vi "Auto Filenames addon.vi"() -> (3 "SubOrdner":string)   [LabVIEW 2020, in "Linearisierung v2.lvlib" / "SpanEinstellungen.lvlib"]
uses:
  SpanEinstellungen.lvlib
  Aktion FGV Post Processing.ctl
  Allgemein/allgemeine Sub-VIs.lvlib
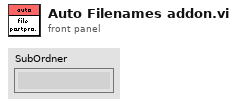
[diagram p1: front panel]
types:
  T1 = typedef "Linearisierung v2.lvlib/SpanEinstellungen.lvlib/Aktion FGV Post Processing.ctl" = enum16{"lesen", "set ref", "init", "reset", "enable", "disable", "filenames", "active", "comp", "filename index", "next", "first", "abort", "show"}
  T2 = typedef "Linearisierung v2.lvlib/SpanEinstellungen.lvlib/Postprocessing_Running_Indices.ctl" = cluster{"active postprocessing SPAN":i32, "active postprocessing SPAN Component":i32, "active postprocessing index":i32}
  T3 = cluster{"active Index Cluster out":T2, "last postprocessing SPAN ":bool}
  T4 = typedef "Pfad-Eingabefeld.ctl" = path
  T5 = cluster{"active SPAN Idx":i32, "Pfad .LIN Datei":T4}[]
  T6 = cluster{"active SPAN Idx":i32, "Pfad .LIN Datei":T4}
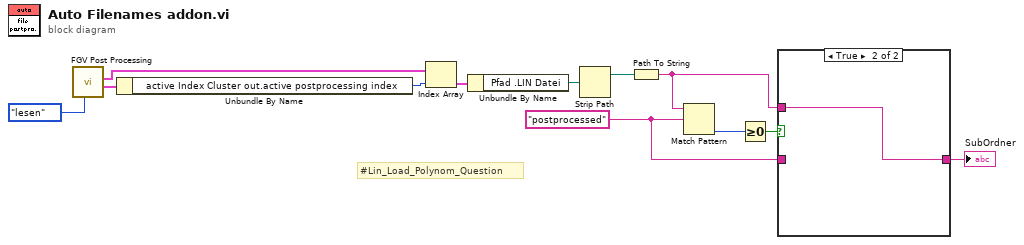
[diagram p0: block diagram]
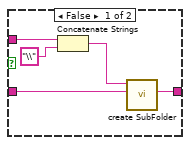
[diagram p2: hidden frame]
diagram:
  w2 = "postprocessed" ("String")
  # "#Lin_Load_Polynom_Question"
  n1 = call "FGV Post Processing.vi"("Aktion"=Aktion_FGV_Post_Processing."lesen") -> ("active Index Cluster out"=w6:T3, "filenemas Cluster Array"=w8:T5)  [unwired: 7 in, 2 out]
  n2 = Unbundle By Name(w6) -> ("active Index Cluster out.active postprocessing index"=w7:i32)
  n3 = Index Array(array=w8, index=w7) -> (element=w9:T6)
  n4 = Unbundle By Name(w9) -> ("Pfad .LIN Datei"=w10:T4)
  n5 = Strip Path(path=w10) -> (stripped path=w11:path)  [unwired: 1 out]
  n6 = Path To String(path=w11) -> (string=w3:string)
  n7 = Match Pattern(string=w3, regular expression=w2) -> (offset past match=w12:i32)  [unwired: 1 in, 3 out]
  n8 = Greater Or Equal To 0?(x=w12) -> (x >= 0?=w4:bool)
  n9 = case shown="True" w4 {
    tunnel: w3 -> [w15 w18]
    tunnel: w2 -> [w14 _]
    tunnel: [w13 w18] -> w1
    frame False {
      n10 = Concatenate Strings(w15, "\\" ("String")) -> (w17:string)
      n11 = call "create SubFolder.vi"("Ordner"=w14, "Pfad"=w17) -> ("SubOrdner"=w13:string)  [unwired: 7 in, 2 out]
    }
    frame True {
    }
  }
  "SubOrdner" <- w1
